vi "GetmsecCounter.vi"(10 "error in (no error)":errorcluster caption="エラー入力（エラーなし）") -> (7 "error out":errorcluster caption="エラー出力", 11 "millisecond timer value":u32)   [LabVIEW 2014]
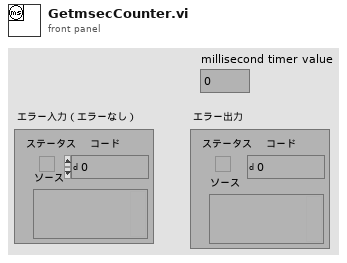
[diagram p1: front panel]
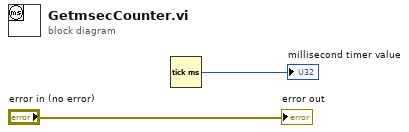
[diagram p0: block diagram]
diagram:
  n1 = Tick Count (ms)() -> (millisecond timer value=→"millisecond timer value":u32)
  "error out" <- "error in (no error)"
